vi "Process_abd_R.vi"(0 "Q_Motor_In":refnum<queue>, 1 "Initialize":bool, 5 "출력 클러스터":T2, 7 "Control param In":T3={"L_velocity"=10000, "L_Power"=0.0, "R_velocity"=10000, "R_Power"=0.0, "T_param_L"={"Onset start"=0.0, "Onset end"=5.0, "Peak start"=10.0, "Release start"=60.0, "slang"=80.0, "Peak end"=58.0}, "T_param_R"={"Onset start"=0.0, "Onset end"=5.0, "Peak start"=10.0, "Release start"=60.0, "slang"=80.0, "Peak end"=58.0}, "Initialize?"=FALSE, "CAN read?"=FALSE, "Optimal count"=0}, 9 "Motor":T1, 11 "에러 입력(에러 없음)":errorcluster, 12 "Param In":T4) -> (3 "R_power_OK":bool, 4 "Q_Motor_Out":refnum<queue>, 8 "GCP_1k_R":sgl, 13 "Control param out":T3, 14 "Param Out":T4, 15 "에러 출력":errorcluster)   [LabVIEW 2019]
uses:
  960d3c6d-78df-4c6d-8941-2c9d2c8cef89.vi
  85e8c586-a1b0-4154-b3af-25e97e6a203b.vi
  <vilib>/numeric/Random Number (Range) I64.vi
  290f23ec-2835-45e2-ad83-d73700e20cec.vi
  d7ad2d91-4bc1-4ce2-a238-38513bee7af7.vi
  020b69f5-43e4-4af2-9fb3-f2528431d2fc.vi
  58df5041-f484-4828-aa8b-3b3581930e24.vi
  3f5fbc32-1fc1-4aa3-983c-412baf48db82.vi
panel:
  in  "Process":T5={"LOAD_CELL_PEAK_L"=[12.0, 8.0], "LOAD_CELL_PEAK_R"=[], "Flag_L"=enum."Release_start", "Flag_R"=enum."Release_start", "Status_PS"="Init", "Q_data"={"Num_L"=0, "Period_L"=0, "GCP_L"=0.0, "Num_R"=0, "Period_R"=0, "GCP_R"=0.0, "FPGA_Data"=[], "L_RUN_OK"=FALSE, "R_RUN_OK"=FALSE, "L_ctrl_start"=FALSE, "R_ctrl_start"=FALSE, "Loop time"=0.0, "Integrated time"=0.0, "Mode"=enum."Negative"}}
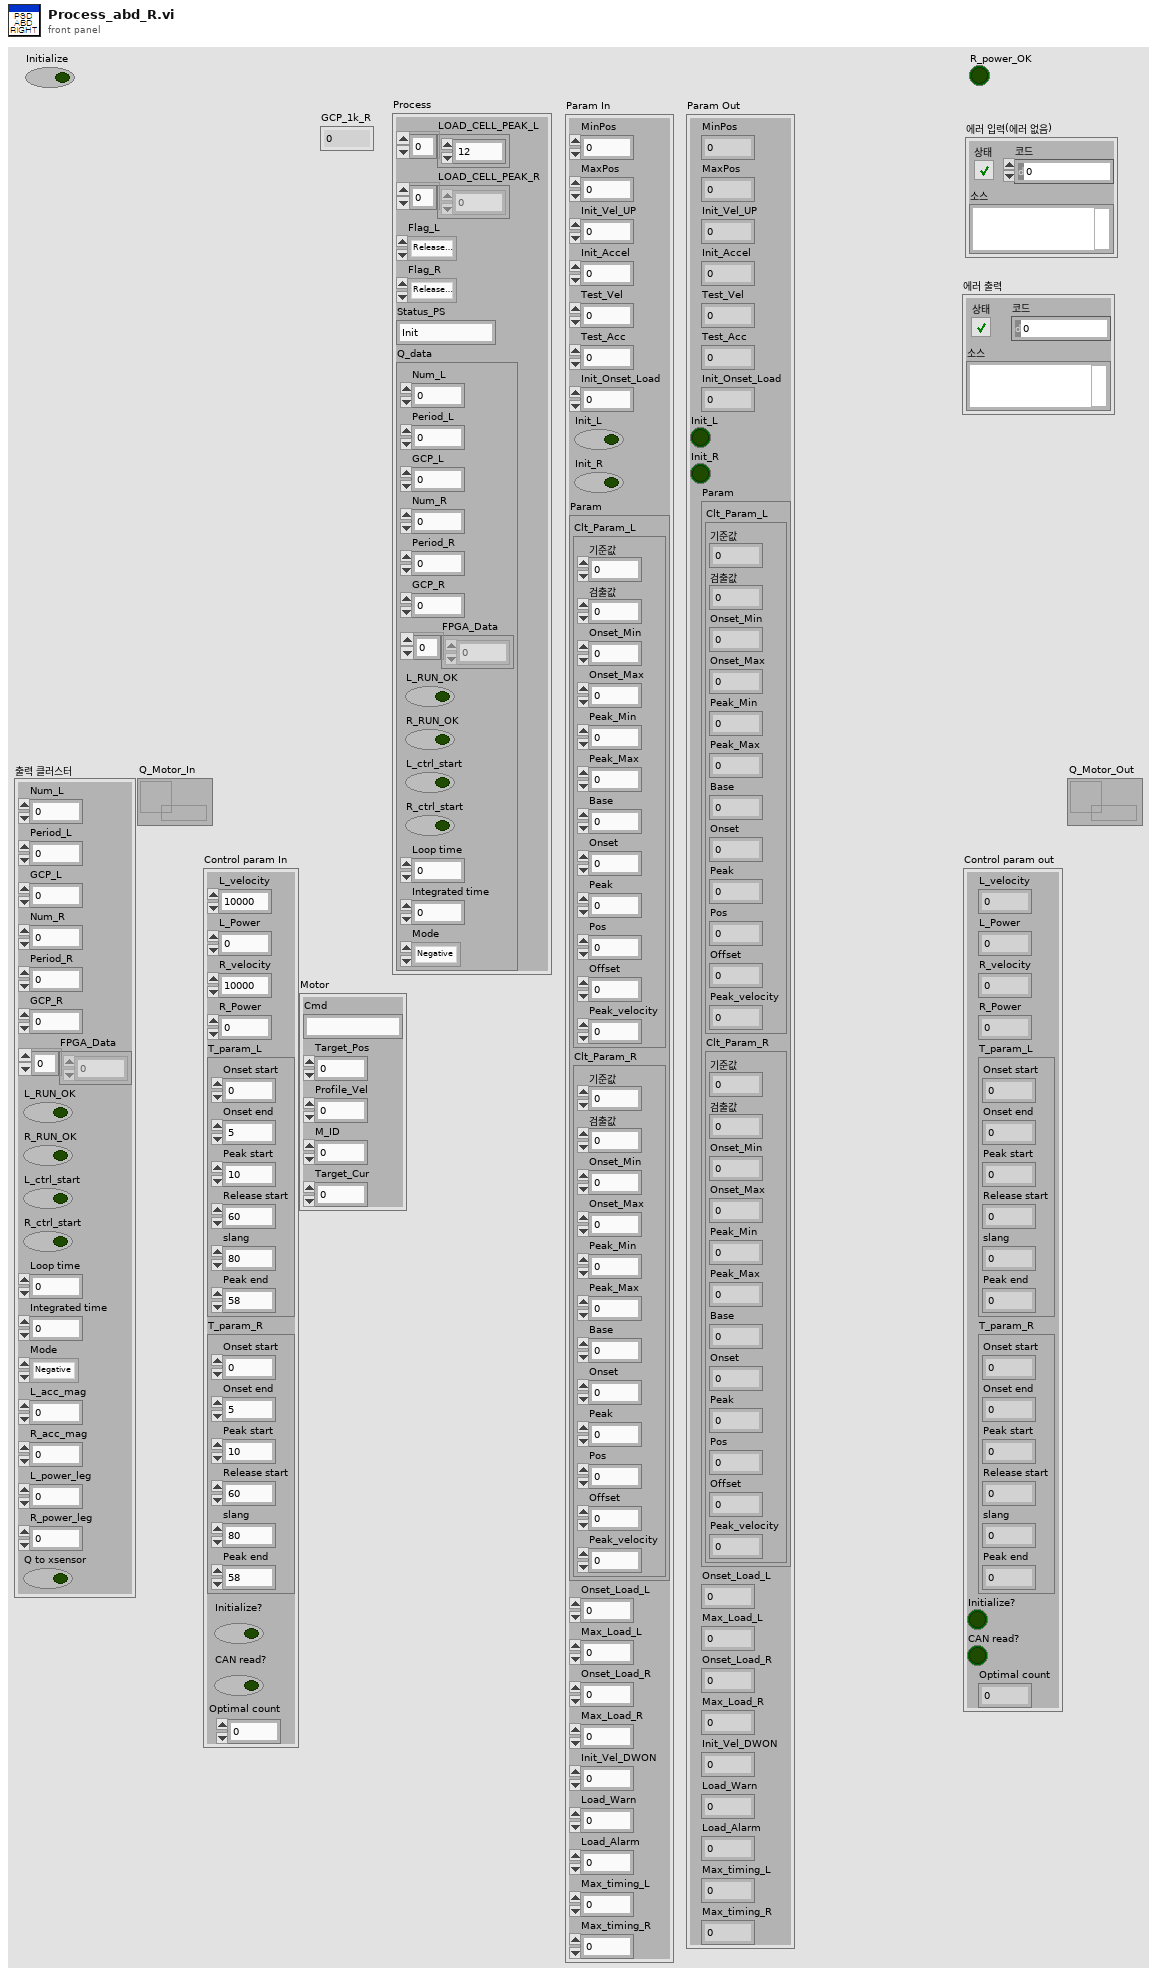
[diagram p1: front panel]
types:
  T1 = cluster{"Cmd":string, "Target_Pos":i32, "Profile_Vel":i32, "M_ID":u8, "Target_Cur":i32}
  T2 = cluster{"Num_L":u32, "Period_L":sgl, "GCP_L":sgl, "Num_R":u32, "Period_R":sgl, "GCP_R":sgl, "FPGA_Data":sgl[], "L_RUN_OK":bool, "R_RUN_OK":bool, "L_ctrl_start":bool, "R_ctrl_start":bool, "Loop time":dbl, "Integrated time":dbl, "Mode":enum16{"Negative", "Positive", "Full"}, "L_acc_mag":sgl, "R_acc_mag":sgl, "L_power_leg":sgl, "R_power_leg":sgl, "Q to xsensor":bool}
  T3 = cluster{"L_velocity":u32, "L_Power":sgl, "R_velocity":u32, "R_Power":sgl, "T_param_L":cluster{"Onset start":sgl, "Onset end":sgl, "Peak start":sgl, "Release start":sgl, "slang":sgl, "Peak end":sgl}, "T_param_R":cluster{"Onset start":sgl, "Onset end":sgl, "Peak start":sgl, "Release start":sgl, "slang":sgl, "Peak end":sgl}, "Initialize?":bool, "CAN read?":bool, "Optimal count":i32}
  T4 = cluster{"MinPos":i32, "MaxPos":i32, "Init_Vel_UP":i32, "Init_Accel":u32, "Test_Vel":i32, "Test_Acc":u32, "Init_Onset_Load":sgl, "Init_L":bool, "Init_R":bool, "Param":cluster{"Clt_Param_L":cluster{"기준값":sgl, "검출값":sgl, "Onset_Min":sgl, "Onset_Max":sgl, "Peak_Min":sgl, "Peak_Max":sgl, "Base":i32, "Onset":i32, "Peak":i32, "Pos":i32, "Offset":sgl, "Peak_velocity":i32}, "Clt_Param_R":cluster{"기준값":sgl, "검출값":sgl, "Onset_Min":sgl, "Onset_Max":sgl, "Peak_Min":sgl, "Peak_Max":sgl, "Base":i32, "Onset":i32, "Peak":i32, "Pos":i32, "Offset":sgl, "Peak_velocity":i32}}, "Onset_Load_L":sgl, "Max_Load_L":sgl, "Onset_Load_R":sgl, "Max_Load_R":sgl, "Init_Vel_DWON":i32, "Load_Warn":sgl, "Load_Alarm":sgl, "Max_timing_L":sgl, "Max_timing_R":sgl}
  T5 = cluster{"LOAD_CELL_PEAK_L":sgl[], "LOAD_CELL_PEAK_R":sgl[], "Flag_L":enum16{"Release_start", "Calculate", "Onset_start", "Peak_start"}, "Flag_R":enum16{"Release_start", "Calculate", "Onset_start", "Peak_start"}, "Status_PS":string, "Q_data":cluster{"Num_L":u32, "Period_L":u32, "GCP_L":sgl, "Num_R":u32, "Period_R":u32, "GCP_R":sgl, "FPGA_Data":sgl[], "L_RUN_OK":bool, "R_RUN_OK":bool, "L_ctrl_start":bool, "R_ctrl_start":bool, "Loop time":dbl, "Integrated time":dbl, "Mode":enum16{"Negative", "Positive", "Full"}}}
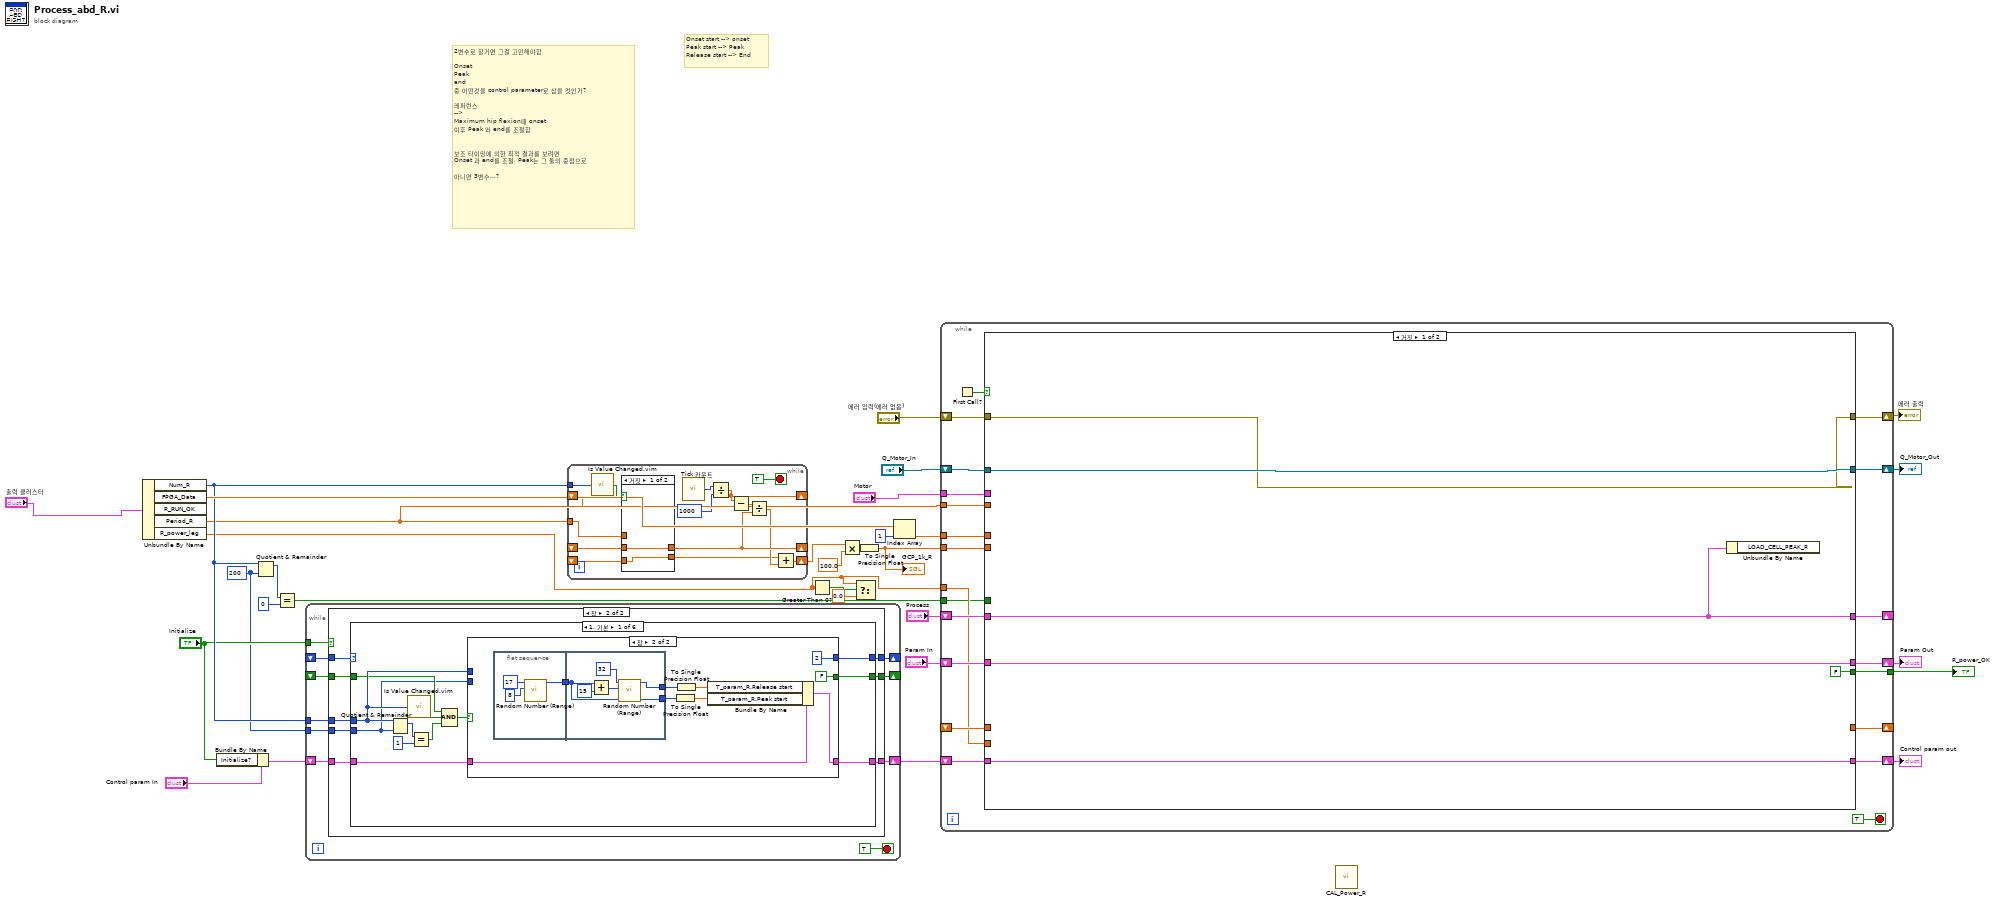
[diagram p0: block diagram]
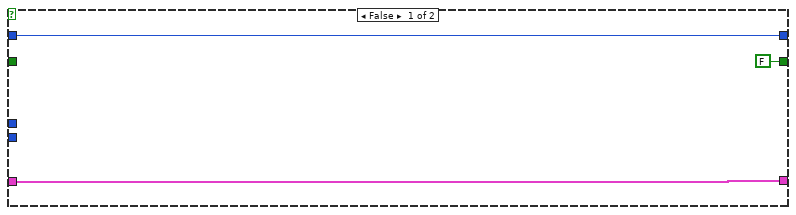
[diagram p2: hidden frame]
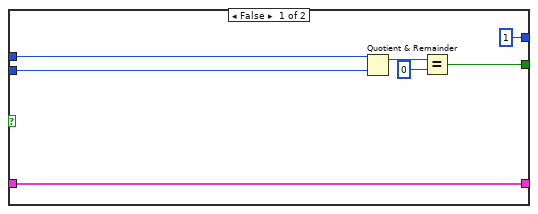
[diagram p3: hidden frame]
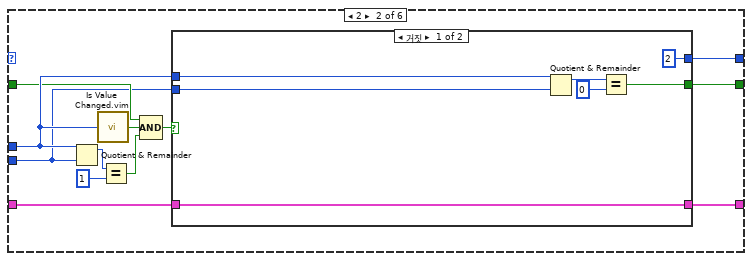
[diagram p4: hidden frame]
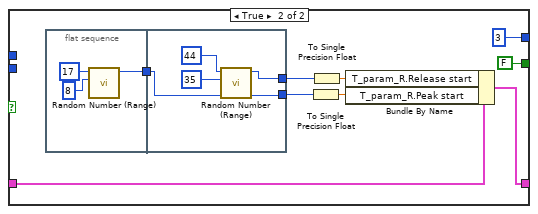
[diagram p5: hidden frame]
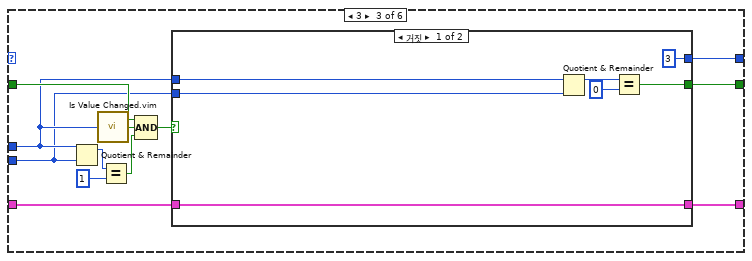
[diagram p6: hidden frame]
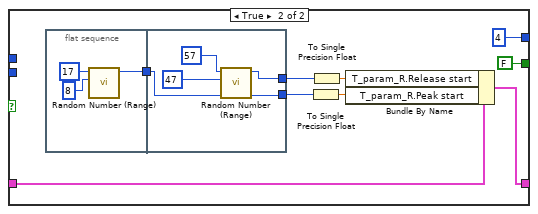
[diagram p7: hidden frame]
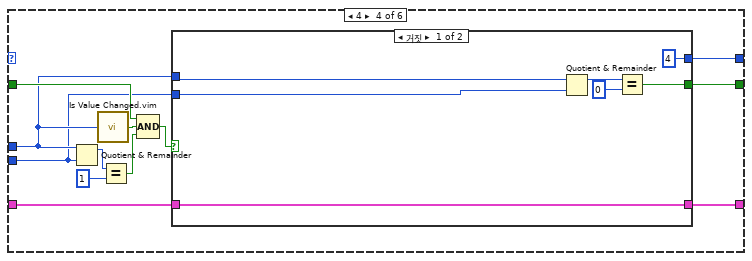
[diagram p8: hidden frame]
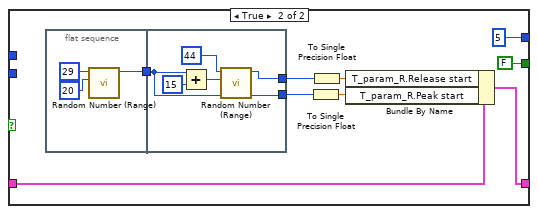
[diagram p9: hidden frame]
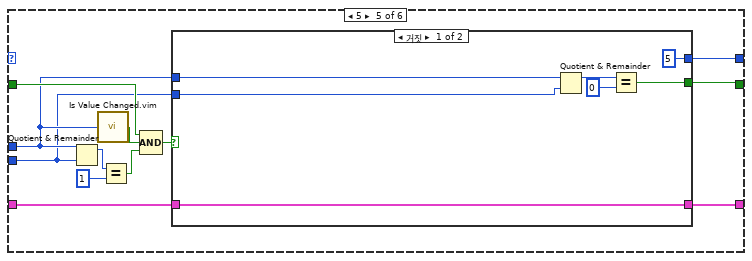
[diagram p10: hidden frame]
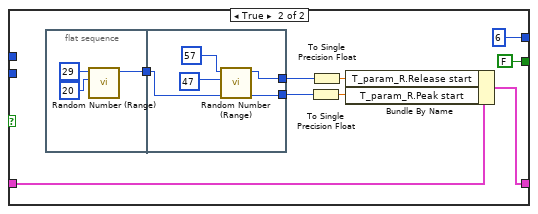
[diagram p11: hidden frame]
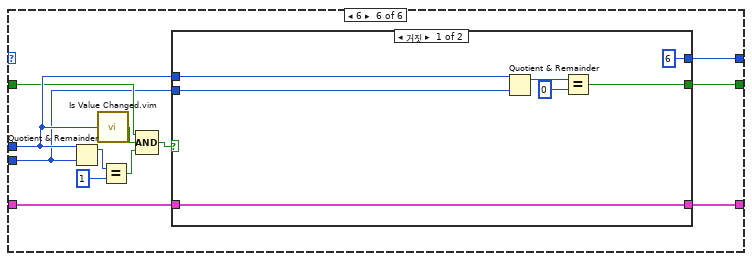
[diagram p12: hidden frame]
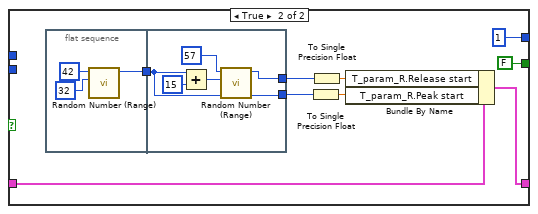
[diagram p13: hidden frame]
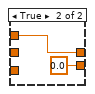
[diagram p14: hidden frame]
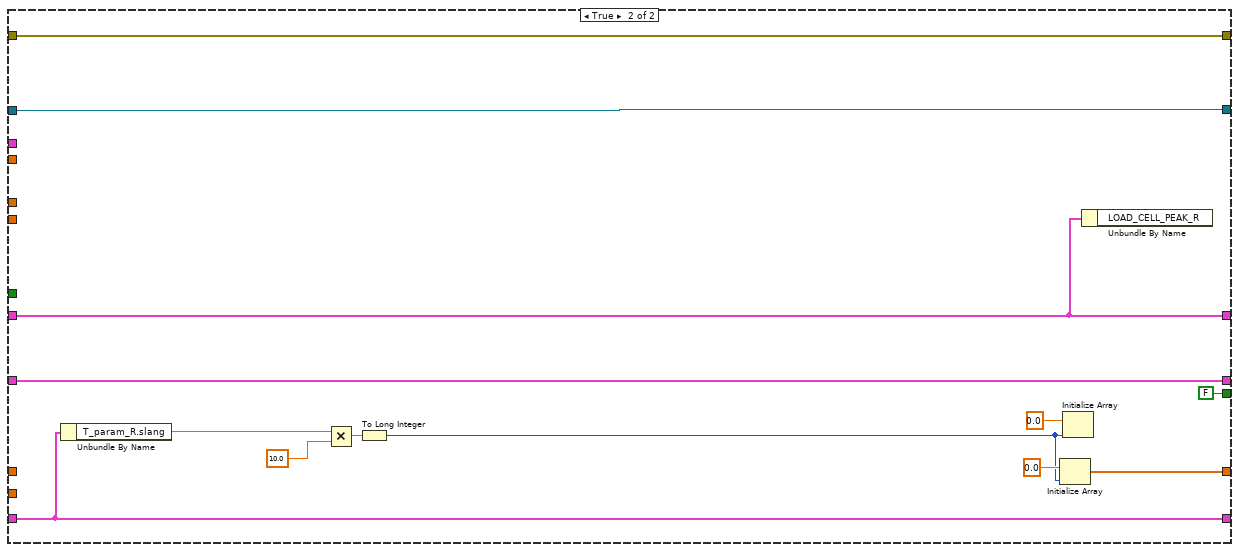
[diagram p15: hidden frame]
diagram:
  w4 = u32 200 ("y")
  # "Onset start --> onset\nPeak start --> Peak\nRelease start --> End"
  # "2변수로 할거면 그걸 고민해야함\n\nOnset\nPeak \nend \n중 어떤것을 control parameter로 삼을 것인가?\n\n레퍼런스\n--> \nMaximum hip flexion때 onset\n이후 Peak 와 end를 조절함\n\n\n보조 타이밍에 의한 최적 결과를 보려면\nOnset 과 end를 조절, Peak는 그 둘의 중점으로\n\n아니면 3변수...?"
  n1 = Unbundle By Name("출력 클러스터") -> ("Num_R"=w16:u32, "FPGA_Data"=w28:sgl[], "Period_R"=w12:sgl, "R_power_leg"=w6:sgl)  [unwired: 1 out]
  n2 = Bundle By Name(cluster="Control param In", "Initialize?"="Initialize") -> (w14:T3)
  n3 = Quotient & Remainder(x=w16, y=w4) -> (x-y*floor(x/y)=w18:u32)  [unwired: 1 out]
  n4 = Equal?(x=w18, y=u32 0) -> (x = y?=w9:bool)
  n5 = while {
    tunnel: w16 -> [w40]
    tunnel: "Initialize" -> [w38]
    shift-right: [w41] -> w19
    shift-left: w14 -> [w39]
    shift-right: [w36] -> _
    shift-left: _ -> [w35]
    shift-right: [w34] -> _
    shift-left: _ -> [w33]
    tunnel: w4 -> [w32]
    stop <- TRUE stop-if-true
    n6 = case shown="참" w38 {
      tunnel: w40 -> [_ w50]
      tunnel: w39 -> [w44 w52]
      tunnel: [w44 w51] -> w41
      tunnel: [w43 w49] -> w36
      tunnel: w35 -> [w43 w48]
      tunnel: [FALSE w47] -> w34
      tunnel: w33 -> [_ w46]
      tunnel: w32 -> [_ w45]
      frame False {
      }
      frame True {
        n7 = case shown="1, 기본" w48 {
          tunnel: w52 -> [w64 w100 w135 w170 w206 w241]
          tunnel: [w63 w99 w134 w169 w205 w240] -> w51
          tunnel: w50 -> [w55 w91 w125 w160 w196 w233]
          tunnel: [w57 w96 w131 w166 w199 w234] -> w49
          tunnel: [w56 w92 w127 w162 w198 w232] -> w47
          tunnel: w46 -> [w54 w90 w126 w161 w197 w231]
          tunnel: w45 -> [w53 w89 w124 w159 w195 w230]
          frame 1, Default {
            n8 = Quotient & Remainder(x=w55, y=w53) -> (x-y*floor(x/y)=w60:u32)  [unwired: 1 out]
            n9 = call "Is Value Changed.vim"("value"=w55) -> ("changed or first call?"=w62:bool)
            n10 = Equal?(x=w60, y=u32 1) -> (x = y?=w58:bool)
            n11 = Compound Arithmetic op=AND ("복합 연산")(w54, w62, w58) -> (w61:bool)
            n12 = case shown="참" w61 {
              tunnel: w64 -> [w71 w77]
              tunnel: [w71 w80] -> w63
              tunnel: [1 2] -> w57
              tunnel: [w67 FALSE] -> w56
              tunnel: w55 -> [w66 _]
              tunnel: w53 -> [w65 _]
              frame False {
                n13 = Quotient & Remainder(x=w66, y=w65) -> (x-y*floor(x/y)=w69:u32)  [unwired: 1 out]
                n14 = Equal?(x=w69, y=u32 0) -> (x = y?=w67:bool)
              }
              frame True {
                n15 = flat-sequence {
                  tunnel: [w81] -> w76
                  tunnel: w76 -> [w84]
                  tunnel: [w85] -> w75
                  tunnel: [w84] -> w74
                  frame #0 {
                    n16 = call-poly <vilib>:"Random Number (Range).vi"("lower bound (-100)"=i64 8 ("lower bound (0)"), "upper bound (100)"=i64 17) -> ("number"=w81:i64)  [unwired: 9 in]
                  }
                  frame #1 {
                    n17 = Add(x=w84, y=i64 15 ("x")) -> (x+y=w88:i64)
                    n18 = call-poly <vilib>:"Random Number (Range).vi"("lower bound (-100)"=w88, "upper bound (100)"=i64 32) -> ("number"=w85:i64)  [unwired: 9 in]
                  }
                }
                n19 = To Single Precision Float(number=w74) -> (single precision float=w78:sgl)
                n20 = To Single Precision Float(number=w75) -> (single precision float=w79:sgl)
                n21 = Bundle By Name(cluster=w77, "T_param_R.Release start"=w79, "T_param_R.Peak start"=w78) -> (w80:T3)
              }
            }
          }
          frame 2 {
            n22 = Quotient & Remainder(x=w91, y=w89) -> (x-y*floor(x/y)=w98:u32)  [unwired: 1 out]
            n23 = call "Is Value Changed.vim"("value"=w91) -> ("changed or first call?"=w95:bool)
            n24 = Equal?(x=w98, y=u32 1) -> (x = y?=w94:bool)
            n25 = Compound Arithmetic op=AND(w90, w95, w94) -> (w93:bool)
            n26 = case shown="거짓" w93 {
              tunnel: w100 -> [w107 w113]
              tunnel: [w107 w116] -> w99
              tunnel: [2 3] -> w96
              tunnel: [w103 FALSE] -> w92
              tunnel: w91 -> [w102 _]
              tunnel: w89 -> [w101 _]
              frame False {
                n27 = Quotient & Remainder(x=w102, y=w101) -> (x-y*floor(x/y)=w105:u32)  [unwired: 1 out]
                n28 = Equal?(x=w105, y=u32 0) -> (x = y?=w103:bool)
              }
              frame True {
                n29 = flat-sequence {
                  tunnel: [w117] -> w112
                  tunnel: w112 -> [w121]
                  tunnel: [w122] -> w111
                  tunnel: [w121] -> w110
                  frame #0 {
                    n30 = call-poly <vilib>:"Random Number (Range).vi"("lower bound (-100)"=i64 8 ("lower bound (0)"), "upper bound (100)"=i64 17) -> ("number"=w117:i64)  [unwired: 9 in]
                  }
                  frame #1 {
                    n31 = call-poly <vilib>:"Random Number (Range).vi"("lower bound (-100)"=i64 35 ("x"), "upper bound (100)"=i64 44) -> ("number"=w122:i64)  [unwired: 9 in]
                  }
                }
                n32 = To Single Precision Float(number=w110) -> (single precision float=w114:sgl)
                n33 = To Single Precision Float(number=w111) -> (single precision float=w115:sgl)
                n34 = Bundle By Name(cluster=w113, "T_param_R.Release start"=w115, "T_param_R.Peak start"=w114) -> (w116:T3)
              }
            }
          }
          frame 3 {
            n35 = Quotient & Remainder(x=w125, y=w124) -> (x-y*floor(x/y)=w133:u32)  [unwired: 1 out]
            n36 = call "Is Value Changed.vim"("value"=w125) -> ("changed or first call?"=w130:bool)
            n37 = Equal?(x=w133, y=u32 1) -> (x = y?=w129:bool)
            n38 = Compound Arithmetic op=AND(w126, w130, w129) -> (w128:bool)
            n39 = case shown="거짓" w128 {
              tunnel: w135 -> [w142 w148]
              tunnel: [w142 w151] -> w134
              tunnel: [3 4] -> w131
              tunnel: [w138 FALSE] -> w127
              tunnel: w125 -> [w137 _]
              tunnel: w124 -> [w136 _]
              frame False {
                n40 = Quotient & Remainder(x=w137, y=w136) -> (x-y*floor(x/y)=w140:u32)  [unwired: 1 out]
                n41 = Equal?(x=w140, y=u32 0) -> (x = y?=w138:bool)
              }
              frame True {
                n42 = flat-sequence {
                  tunnel: [w152] -> w147
                  tunnel: w147 -> [w156]
                  tunnel: [w157] -> w146
                  tunnel: [w156] -> w145
                  frame #0 {
                    n43 = call-poly <vilib>:"Random Number (Range).vi"("lower bound (-100)"=i64 8 ("lower bound (0)"), "upper bound (100)"=i64 17) -> ("number"=w152:i64)  [unwired: 9 in]
                  }
                  frame #1 {
                    n44 = call-poly <vilib>:"Random Number (Range).vi"("lower bound (-100)"=i64 47 ("x"), "upper bound (100)"=i64 57) -> ("number"=w157:i64)  [unwired: 9 in]
                  }
                }
                n45 = To Single Precision Float(number=w145) -> (single precision float=w149:sgl)
                n46 = To Single Precision Float(number=w146) -> (single precision float=w150:sgl)
                n47 = Bundle By Name(cluster=w148, "T_param_R.Release start"=w150, "T_param_R.Peak start"=w149) -> (w151:T3)
              }
            }
          }
          frame 4 {
            n48 = Quotient & Remainder(x=w160, y=w159) -> (x-y*floor(x/y)=w168:u32)  [unwired: 1 out]
            n49 = call "Is Value Changed.vim"("value"=w160) -> ("changed or first call?"=w164:bool)
            n50 = Equal?(x=w168, y=u32 1) -> (x = y?=w165:bool)
            n51 = Compound Arithmetic op=AND(w161, w164, w165) -> (w163:bool)
            n52 = case shown="거짓" w163 {
              tunnel: w170 -> [w177 w183]
              tunnel: [w177 w186] -> w169
              tunnel: [4 5] -> w166
              tunnel: [w173 FALSE] -> w162
              tunnel: w160 -> [w172 _]
              tunnel: w159 -> [w171 _]
              frame False {
                n53 = Quotient & Remainder(x=w172, y=w171) -> (x-y*floor(x/y)=w175:u32)  [unwired: 1 out]
                n54 = Equal?(x=w175, y=u32 0) -> (x = y?=w173:bool)
              }
              frame True {
                n55 = flat-sequence {
                  tunnel: [w187] -> w182
                  tunnel: w182 -> [w190]
                  tunnel: [w191] -> w181
                  tunnel: [w190] -> w180
                  frame #0 {
                    n56 = call-poly <vilib>:"Random Number (Range).vi"("lower bound (-100)"=i64 20 ("lower bound (0)"), "upper bound (100)"=i64 29) -> ("number"=w187:i64)  [unwired: 9 in]
                  }
                  frame #1 {
                    n57 = Add(x=w190, y=i64 15 ("x")) -> (x+y=w194:i64)
                    n58 = call-poly <vilib>:"Random Number (Range).vi"("lower bound (-100)"=w194, "upper bound (100)"=i64 44) -> ("number"=w191:i64)  [unwired: 9 in]
                  }
                }
                n59 = To Single Precision Float(number=w180) -> (single precision float=w184:sgl)
                n60 = To Single Precision Float(number=w181) -> (single precision float=w185:sgl)
                n61 = Bundle By Name(cluster=w183, "T_param_R.Release start"=w185, "T_param_R.Peak start"=w184) -> (w186:T3)
              }
            }
          }
          frame 5 {
            n62 = Quotient & Remainder(x=w196, y=w195) -> (x-y*floor(x/y)=w202:u32)  [unwired: 1 out]
            n63 = call "Is Value Changed.vim"("value"=w196) -> ("changed or first call?"=w204:bool)
            n64 = Equal?(x=w202, y=u32 1) -> (x = y?=w200:bool)
            n65 = Compound Arithmetic op=AND ("복합 연산")(w197, w204, w200) -> (w203:bool)
            n66 = case shown="거짓" w203 {
              tunnel: w206 -> [w213 w219]
              tunnel: [w213 w222] -> w205
              tunnel: [5 6] -> w199
              tunnel: [w209 FALSE] -> w198
              tunnel: w196 -> [w208 _]
              tunnel: w195 -> [w207 _]
              frame False {
                n67 = Quotient & Remainder(x=w208, y=w207) -> (x-y*floor(x/y)=w211:u32)  [unwired: 1 out]
                n68 = Equal?(x=w211, y=u32 0) -> (x = y?=w209:bool)
              }
              frame True {
                n69 = flat-sequence {
                  tunnel: [w223] -> w218
                  tunnel: w218 -> [w227]
                  tunnel: [w228] -> w217
                  tunnel: [w227] -> w216
                  frame #0 {
                    n70 = call-poly <vilib>:"Random Number (Range).vi"("lower bound (-100)"=i64 20 ("lower bound (0)"), "upper bound (100)"=i64 29) -> ("number"=w223:i64)  [unwired: 9 in]
                  }
                  frame #1 {
                    n71 = call-poly <vilib>:"Random Number (Range).vi"("lower bound (-100)"=i64 47 ("x"), "upper bound (100)"=i64 57) -> ("number"=w228:i64)  [unwired: 9 in]
                  }
                }
                n72 = To Single Precision Float(number=w216) -> (single precision float=w220:sgl)
                n73 = To Single Precision Float(number=w217) -> (single precision float=w221:sgl)
                n74 = Bundle By Name(cluster=w219, "T_param_R.Release start"=w221, "T_param_R.Peak start"=w220) -> (w222:T3)
              }
            }
          }
          frame 6 {
            n75 = Quotient & Remainder(x=w233, y=w230) -> (x-y*floor(x/y)=w237:u32)  [unwired: 1 out]
            n76 = call "Is Value Changed.vim"("value"=w233) -> ("changed or first call?"=w239:bool)
            n77 = Equal?(x=w237, y=u32 1) -> (x = y?=w235:bool)
            n78 = Compound Arithmetic op=AND ("복합 연산")(w231, w239, w235) -> (w238:bool)
            n79 = case shown="거짓" w238 {
              tunnel: w241 -> [w248 w254]
              tunnel: [w248 w257] -> w240
              tunnel: [6 1] -> w234
              tunnel: w233 -> [w244 _]
              tunnel: [w243 FALSE] -> w232
              tunnel: w230 -> [w242 _]
              frame False {
                n80 = Quotient & Remainder(x=w244, y=w242) -> (x-y*floor(x/y)=w246:u32)  [unwired: 1 out]
                n81 = Equal?(x=w246, y=u32 0) -> (x = y?=w243:bool)
              }
              frame True {
                n82 = flat-sequence {
                  tunnel: [w258] -> w253
                  tunnel: w253 -> [w261]
                  tunnel: [w262] -> w252
                  tunnel: [w261] -> w251
                  frame #0 {
                    n83 = call-poly <vilib>:"Random Number (Range).vi"("lower bound (-100)"=i64 32 ("lower bound (0)"), "upper bound (100)"=i64 42) -> ("number"=w258:i64)  [unwired: 9 in]
                  }
                  frame #1 {
                    n84 = Add(x=w261, y=i64 15 ("x")) -> (x+y=w265:i64)
                    n85 = call-poly <vilib>:"Random Number (Range).vi"("lower bound (-100)"=w265, "upper bound (100)"=i64 57) -> ("number"=w262:i64)  [unwired: 9 in]
                  }
                }
                n86 = To Single Precision Float(number=w251) -> (single precision float=w255:sgl)
                n87 = To Single Precision Float(number=w252) -> (single precision float=w256:sgl)
                n88 = Bundle By Name(cluster=w254, "T_param_R.Release start"=w256, "T_param_R.Peak start"=w255) -> (w257:T3)
              }
            }
          }
        }
      }
    }
  }
  n89 = while {
    shift-right: [w278] -> _
    shift-left: _ -> [w279]
    shift-right: [w276] -> w24
    shift-left: _ -> [w275]
    shift-right: [w269] -> _
    shift-left: _ -> [w272]
    tunnel: w12 -> [w268]
    tunnel: w16 -> [w267]
    stop <- TRUE stop-if-true
    n90 = call "Is Value Changed.vim"("value"=w267) -> ("changed or first call?"=w266:bool)
    n91 = case shown="거짓" w266 {
      tunnel: w268 -> [_ w284]
      tunnel: [w282 w284] -> w278
      tunnel: w279 -> [w282 _]
      tunnel: w275 -> [w281 _]
      tunnel: [w281 0.0] -> w274
      frame False {
      }
      frame True {
      }
    }
    n92 = call "Tick 카운트"() -> ("Tick Count(uSec)"=w271:u32)
    n93 = Divide(x=w271, y=u32 1000) -> (x/y=w269:dbl)
    n94 = Subtract(x=w269, y=w272) -> (x-y=w273:dbl)
    n95 = Divide(x=w273, y=w278) -> (x/y=w277:dbl)
    n96 = Add(x=w274, y=w277) -> (x+y=w276:dbl)
  }
  n97 = Greater Than 0?(x=w6) -> (x > 0?=w8:bool)
  n98 = Multiply(x=w24, y=100.0) -> (x*y=w25:dbl)
  n99 = Select(t=w6, s=w8, f=sgl 0.0 ("하위 리미트")) -> ()  [unwired: 1 out]
  n100 = To Single Precision Float(number=w25) -> (single precision float=w23:sgl)
  "GCP_1k_R" <- w23
  n101 = Index Array(array=w28, index=1 ("인덱스")) -> (element=w26:sgl)
  n102 = while {
    tunnel: w12 -> [w301]
    tunnel: "Motor" -> [w298]
    tunnel: w26 -> [w296]
    tunnel: w23 -> [w295]
    shift-right: [w304] -> _
    shift-left: "Process" -> [w303]
    shift-right: [w305] -> w31
    shift-left: "에러 입력(에러 없음)" -> [w299]
    shift-right: [w302] -> w2
    shift-left: "Q_Motor_In" -> [w297]
    shift-right: [w300] -> w21
    shift-left: "Param In" -> [w294]
    shift-right: [w291] -> _
    shift-left: _ -> [w290]
    tunnel: w6 -> [w289]
    shift-right: [w288] -> w10
    shift-left: w19 -> [w287]
    tunnel: [w286] -> w20
    tunnel: w9 -> [w285]
    stop <- TRUE stop-if-true
    n103 = First Call?() -> (First Call?: T/F=w293:bool)
    n104 = case shown="거짓" w293 {
      tunnel: w294 -> [w310 w321]
      tunnel: w295 -> [_ _]
      tunnel: w296 -> [_ _]
      tunnel: w297 -> [w312 w325]
      tunnel: w298 -> [_ _]
      tunnel: [w312 w325] -> w302
      tunnel: w299 -> [w311 w324]
      tunnel: [w311 w324] -> w305
      tunnel: [w310 w321] -> w300
      tunnel: w301 -> [_ _]
      tunnel: w303 -> [w309 w323]
      tunnel: [w309 w323] -> w304
      tunnel: [_ w315] -> w291
      tunnel: w290 -> [_ _]
      tunnel: w289 -> [_ _]
      tunnel: [w308 w314] -> w288
      tunnel: w287 -> [w308 w314]
      tunnel: [FALSE ("R_power_OK") FALSE ("R_power_OK")] -> w286
      tunnel: w285 -> [_ _]
      frame False {
        n105 = Unbundle By Name(w309) -> ("LOAD_CELL_PEAK_R"=w306:sgl[])
      }
      frame True {
        n106 = Unbundle By Name(w314) -> ("T_param_R.slang"=w320:sgl)
        n107 = Multiply(x=w320, y=sgl 10.0) -> (x*y=w318:sgl)
        n108 = To Long Integer(number=w318) -> (32bit integer=w316:i32)
        n109 = Initialize Array(sgl 0.0 ("원소"), w316) -> (w315:sgl[])
        n110 = Initialize Array(sgl 0.0 ("원소"), w316) -> (w326:sgl[])
        n111 = Unbundle By Name(w323) -> ("LOAD_CELL_PEAK_R"=w322:sgl[])
      }
    }
  }
  "에러 출력" <- w31
  "Param Out" <- w21
  "R_power_OK" <- w20
  "Control param out" <- w10
  "Q_Motor_Out" <- w2
  n112 = call "CAL_Power_R.vi"() -> ()  [unwired: 7 in, 4 out]
